vi "Read Scope.vi"(11 "Attribute in":refnum<class "Attribute.lvclass">) -> (2 "Scope":T1, 3 "Attribute out":refnum<class "Attribute.lvclass">)   [LabVIEW 2021, in "smo.lvlib" / "Attribute.lvclass"]
uses:
  Attribute.lvclass
  Definitions/def.SMO/Scope -- Enum.ctl
  Attribute.lvclass/Attribute.ctl
  Definitions/def.SMO/def.SMO.lvclass
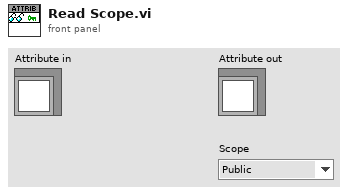
[diagram p1: front panel]
types:
  T1 = typedef "smo.lvlib/def.SMO.lvclass/Scope -- Enum.ctl" = enum16{"Public", "Protected", "Private"}
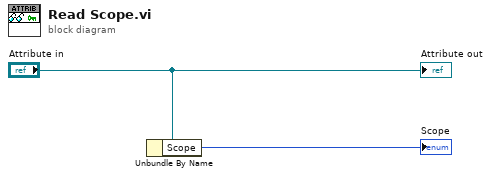
[diagram p0: block diagram]
diagram:
  n1 = Unbundle By Name("Attribute in") -> ("Scope"=→"Scope":T1)
  "Attribute out" <- "Attribute in"
